vi "XYZ-IRC_Api.vi"(3 "精準度":dbl=30.0, 4 "ExitRange":dbl=0.08, 5 "加速度":dbl=800.0, 6 "目標電壓":dbl[](array[numeric])=[2.00487, 1.87997, 1.94422, 1.88569, 1.82844, 1.91098, 1.88335, 2.08625], 7 "最高速":dbl=1150.0, 8 "Error":errorcluster, 9 "副邊校正":T1(ring)=enum."無", 10 "主編校正":enum16{"前", "後", "オ", "右", "無"}(ring)=enum."無", 11 "X-Y-Z移動":dbl[](array[numeric])=[0.0, 0.0, 0.0]) -> (0 "Error Out":errorcluster)   [LabVIEW 2019]
uses:
  <vilib>/Platform/TimedLoop/XDataNode/timing_clust.ctl
  <vilib>/Platform/TimedLoop/XDataNode/nitl_modes.ctl
  <vilib>/Platform/TimedLoop/XDataNode/wakeup.ctl
  <vilib>/addons/control/pid/pid.llb/PID (DBL Array).vi
  <vilib>/platform/TimedLoop/XDataNode/XDataNode.xnode
  <vilib>/Platform/TimedLoop/XDataNode/XDNodeRunTimeDep.lvlib
  <vilib>/addons/control/pid/NI_PID_pid.lvlib
panel:
  in  "Stop":bool
  out "三角形?":bool
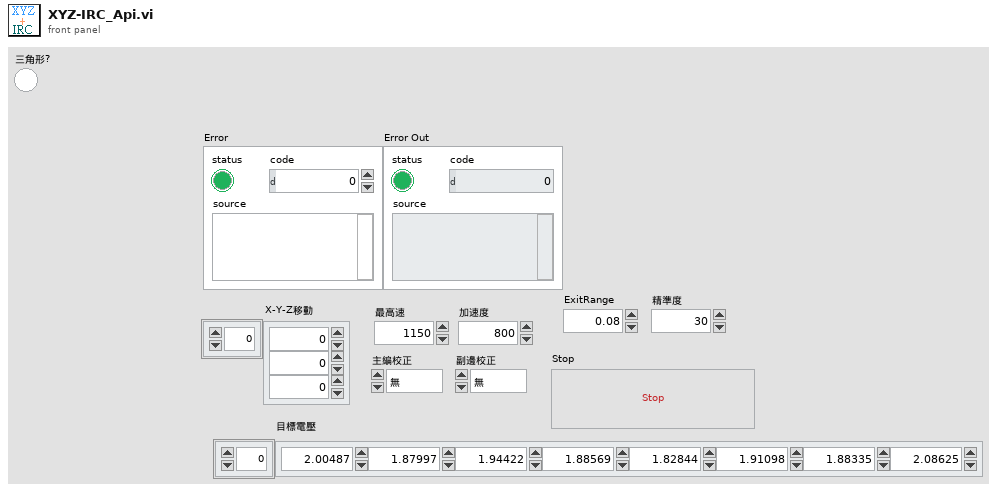
[diagram p1: front panel]
types:
  T1 = enum16{"前", "後", "オ", "右", "無", "0", "1", "2", "3", "4", "5", "6", "7"}
  T2 = cluster{"proportional gain (Kc)":dbl, "integral time (Ti, min)":dbl, "derivative time (Td, min)":dbl}[]
  T3 = typedef "XDNodeRunTimeDep.lvlib/timing_clust.ctl" = cluster{"Expected End [f-1]":u64, "Actual End [f-1]":u64, "Finished Late? [f-1]":bool, "Expected End [i-1]":u64, "Actual End [i-1]":u64, "Finished Late? [i-1]":bool, "Expected Start [i]":u64, "Actual Start [i]":u64, "Expected Start [f]":u64, "Actual Start [f]":u64, "Source Name":string, "Structure Name":string, "Period":i64, "Deadline":i64, "Offset":i64, "Start":i64, "Priority":i32, "Timeout":i32, "Mode":T4, "Wakeup Reason":T5, "Error":errorcluster, "Source Type":string, "Secondary Source Type":string, "Global End Time":u64, "Global Start Time":u64, "Frame Duration":u64, "Iteration Duration":u64, "Assigned CPU":i32, "I/O Scan Engine Mode":u32}
  T4 = typedef "XDNodeRunTimeDep.lvlib/nitl_modes.ctl" = enum32{"No Change", "Process missed periods, maintain original phase", "Discard missed periods, maintain original phase", "Process missed periods, ignore original phase", "Discard missed periods, ignore original phase"}
  T5 = typedef "XDNodeRunTimeDep.lvlib/wakeup.ctl" = enum32{"Normal", "Aborted", "Asynchronous wakeup", "Timing source error", "Timed loop error", "Timeout"}
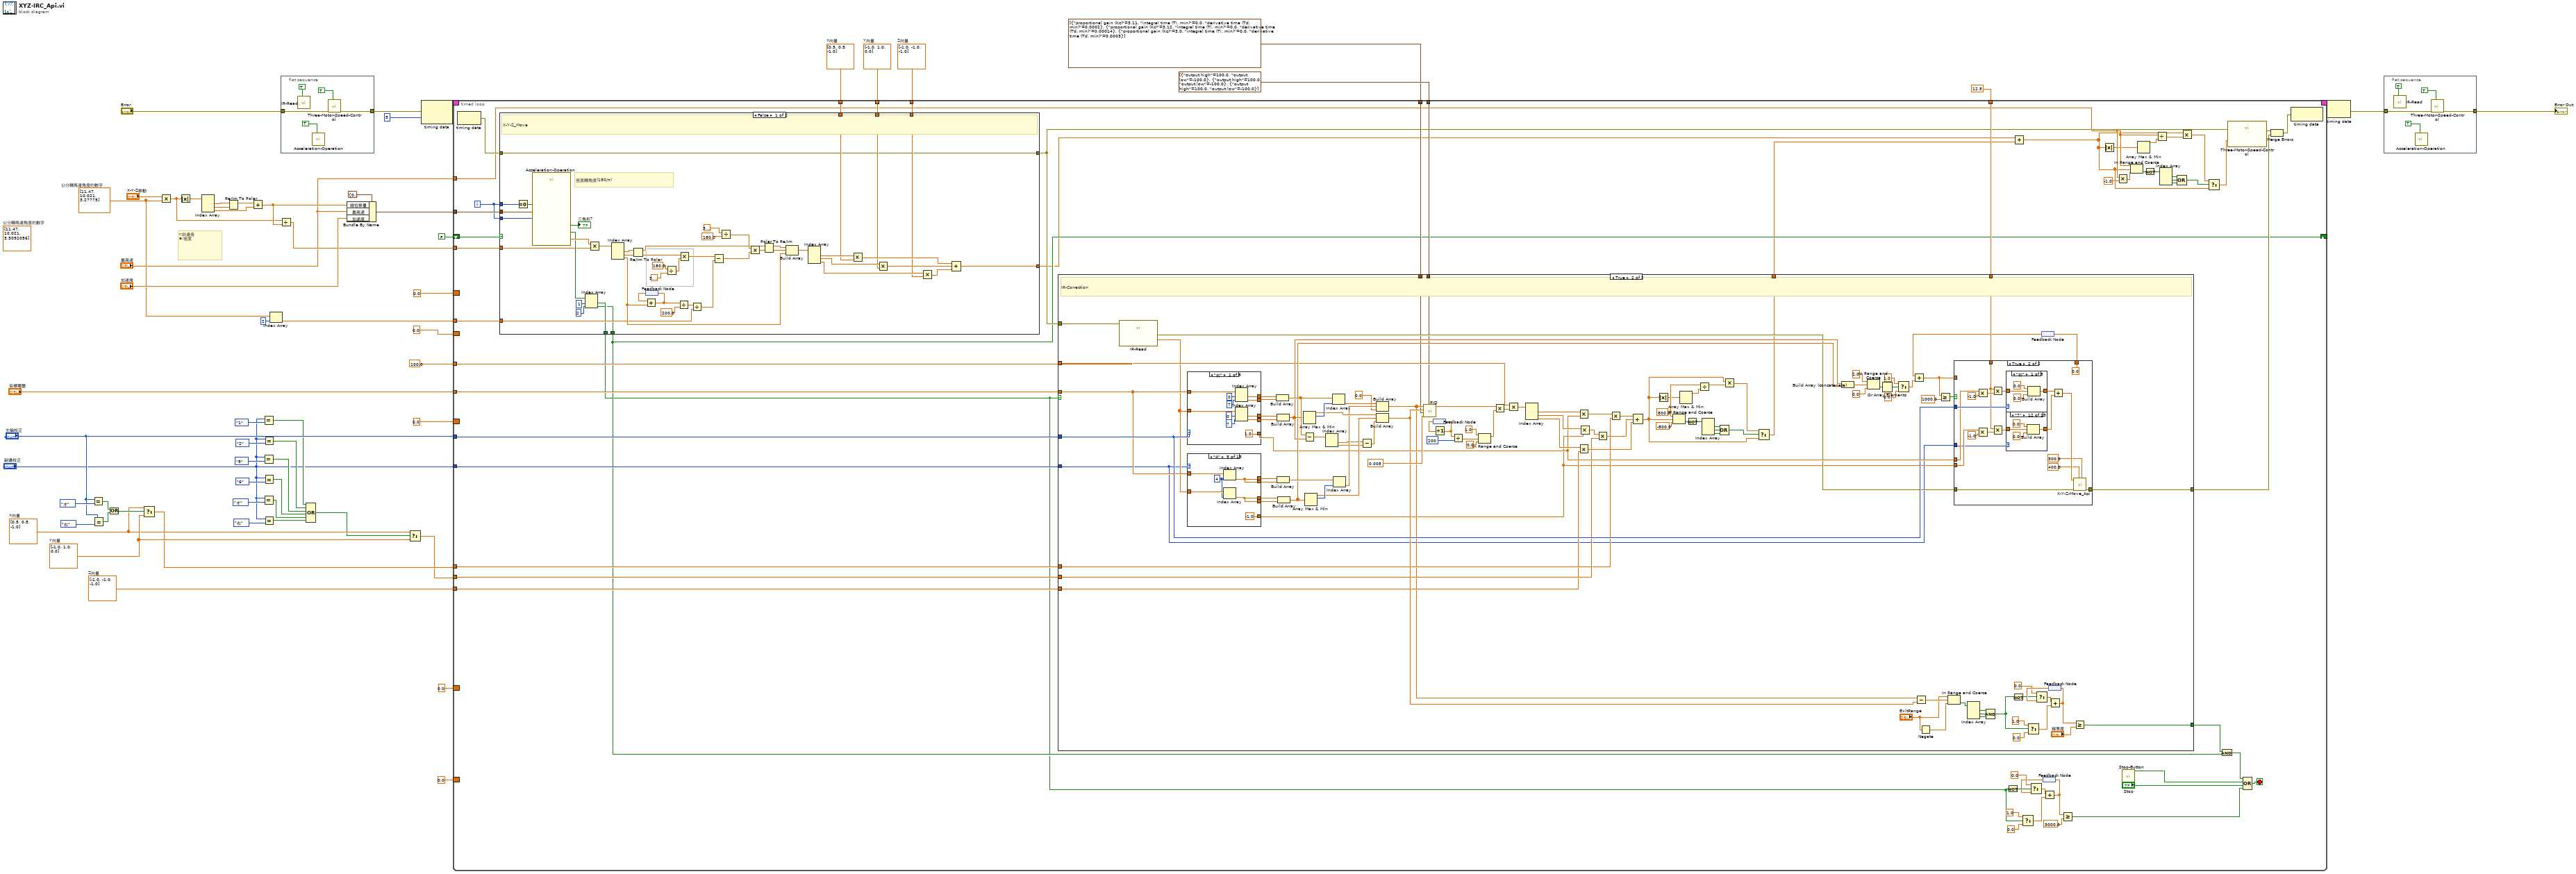
[diagram p0: block diagram]
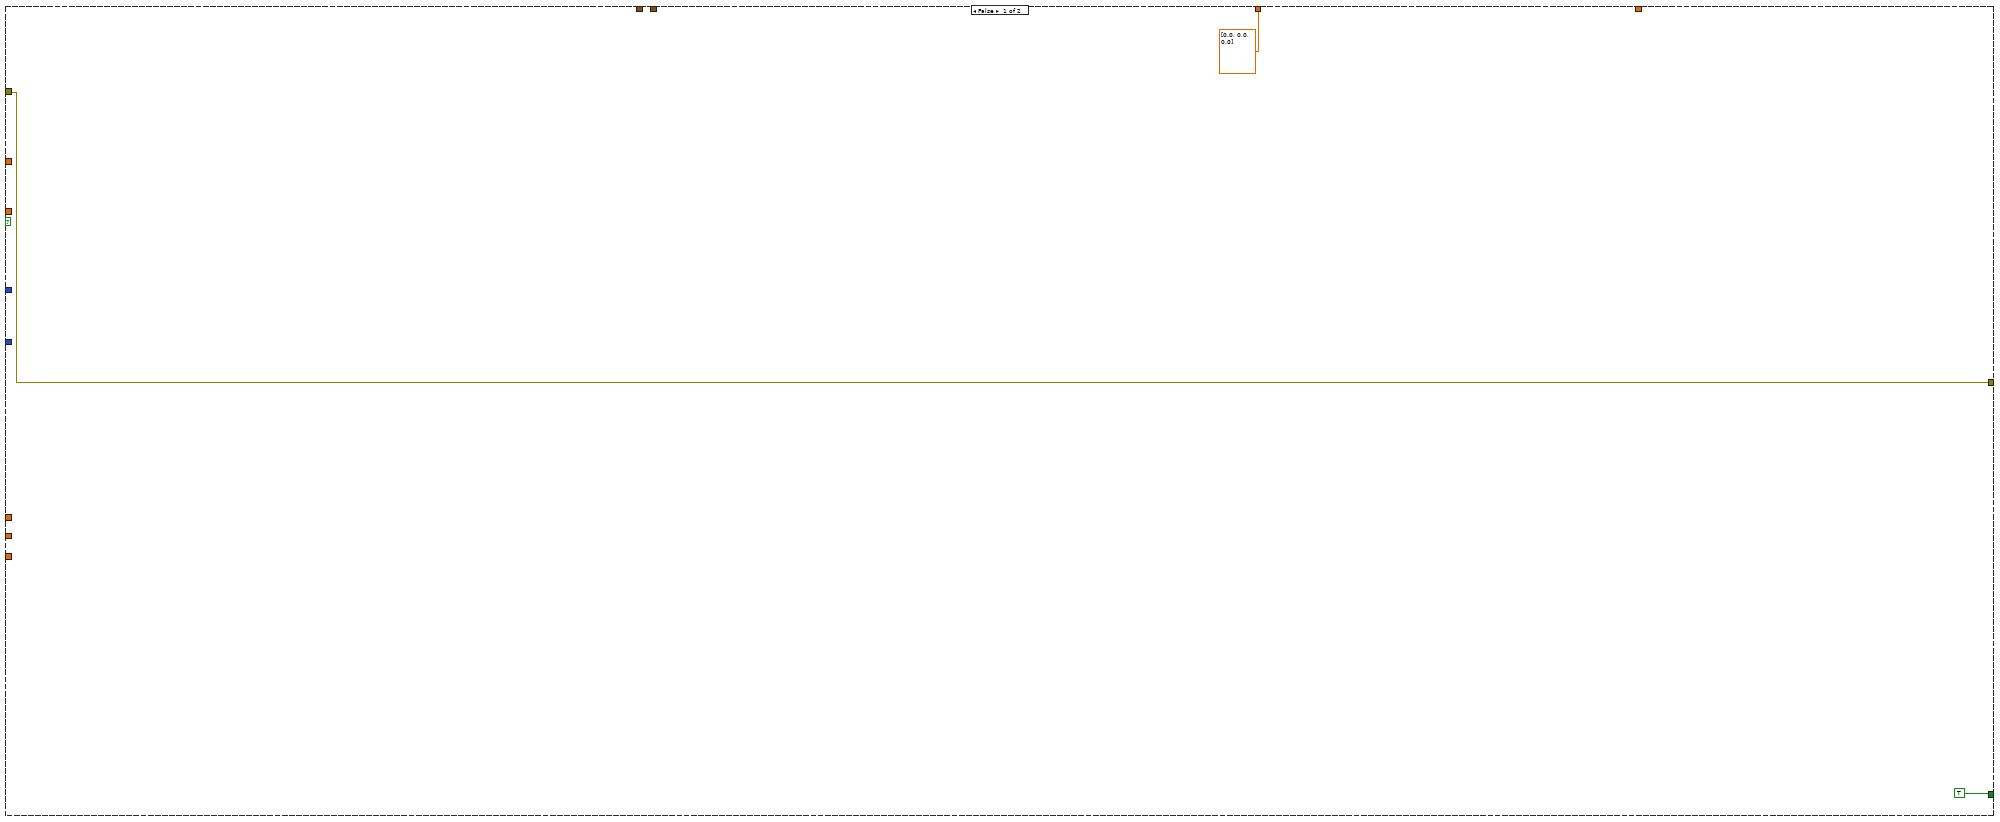
[diagram p2: hidden frame]
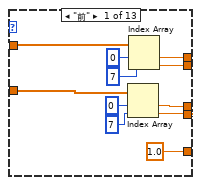
[diagram p3: hidden frame]
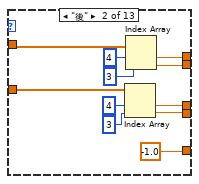
[diagram p4: hidden frame]
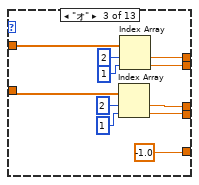
[diagram p5: hidden frame]
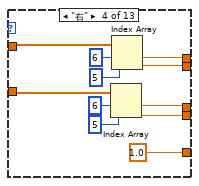
[diagram p6: hidden frame]
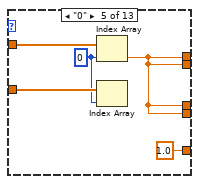
[diagram p7: hidden frame]
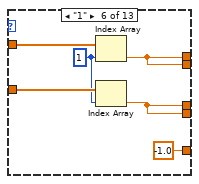
[diagram p8: hidden frame]
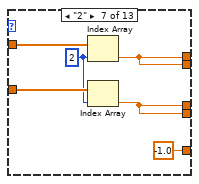
[diagram p9: hidden frame]
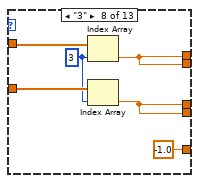
[diagram p10: hidden frame]
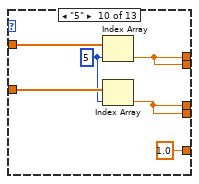
[diagram p11: hidden frame]
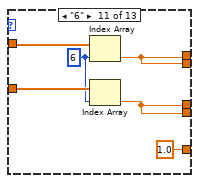
[diagram p12: hidden frame]
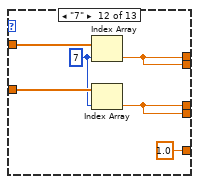
[diagram p13: hidden frame]
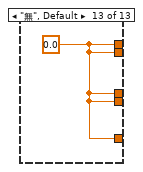
[diagram p14: hidden frame]
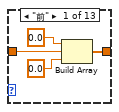
[diagram p16: hidden frame]
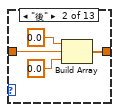
[diagram p17: hidden frame]
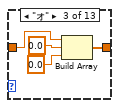
[diagram p18: hidden frame]
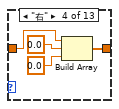
[diagram p19: hidden frame]
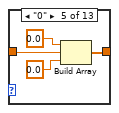
[diagram p20: hidden frame]
diagram:
  w25 = dbl[] [-1.0, -1.0, -1.0]  # Z向量
  w36 = dbl[] [-1.0, 1.0, 0.0]  # Y向量
  w35 = dbl[] [0.5, 0.5, -1.0]  # X向量
  w41 = dbl[] [-1.0, -1.0, -1.0]  # Z向量
  w42 = dbl[] [-1.0, 1.0, 0.0]  # Y向量
  w43 = dbl[] [0.5, 0.5, -1.0]  # X向量
  (unwired) dbl[] [11.47, 10.021, 3.3092056]  # 公分轉馬達角度的數字
  w49 = dbl[] [11.47, 10.021, 3.27775]  # 公分轉馬達角度的數字
  # "r:斜邊長\ne:徑度"
  n1 = Equal?(x="主編校正", y=enum16{"前", "後", "オ", "右", "無"}."オ") -> (x = y?=w38:bool)
  n2 = Equal?(x="主編校正", y=enum16{"前", "後", "オ", "右", "無"}."右") -> (x = y?=w39:bool)
  n3 = Or(x=w38, y=w39) -> (x .or. y?=w37:bool)
  n4 = Select(t=w35, s=w37, f=w36) -> (s? t:f=w27:dbl[])
  n5 = Multiply(x="X-Y-Z移動", y=w49) -> (x*y=w50:dbl[])
  n6 = Absolute Value(x=w50) -> (abs(x)=w58:dbl[])
  n7 = Index Array(array=w58) -> (element #1=w54:dbl, element #2=w59:dbl, element #3=w55:dbl)  [unwired: 3 in]
  n8 = Re/Im To Polar(2:w59, 3:w54) -> (1:w56:dbl)  [unwired: 1 out]
  n9 = Add(x=w56, y=w55) -> (x+y=w51:dbl)
  n10 = Equal?(x="副邊校正", y=T1."1") -> (x = y?=w5:bool)
  n11 = Equal?(x="副邊校正", y=T1."5") -> (x = y?=w4:bool)
  n12 = Equal?(x="副邊校正", y=T1."オ") -> (x = y?=w8:bool)
  n13 = Equal?(x="副邊校正", y=T1."2") -> (x = y?=w6:bool)
  n14 = Equal?(x="副邊校正", y=T1."6") -> (x = y?=w7:bool)
  n15 = Equal?(x="副邊校正", y=T1."右") -> (x = y?=w9:bool)
  n16 = Index Array(array=w49, index=2) -> (element=w45:dbl)
  n17 = Divide(x=w50, y=w51) -> (x/y=w46:dbl[])
  n18 = flat-sequence {
    tunnel: "Error" -> [w66]
    tunnel: [w65] -> w40
    frame #0 {
      n19 = call "IR-Read.vi"("Reset"=TRUE) -> ()  [unwired: 9 in, 2 out]
      n20 = call "Acceleration-Operation.vi"("Reset"=TRUE) -> ()  [unwired: 8 in, 3 out]
      n21 = call "Three-Motor-Speed-Control.vi"("Reset"=TRUE, "Error In"=w66) -> ("Error Out"=w65:errorcluster)  [unwired: 9 in]
    }
  }
  n22 = Compound Arithmetic op=OR(w5, w6, w4, w7, w8, w9) -> (w2:bool)
  n23 = Bundle By Name(cluster=cluster{"總位移量":dbl, "最高速":dbl, "加速度":dbl} {"總位移量"=0.0, "最高速"=0.0, "加速度"=0.0} ("計算設置"), "總位移量"=w51, "最高速"="最高速", "加速度"="加速度") -> (w47:cluster{"總位移量":dbl, "最高速":dbl, "加速度":dbl})
  n24 = Select(t=w35, s=w2, f=w36) -> (s? t:f=w26:dbl[])
  n25 = node-c288(w40, i64 5 ("Period")) -> (w62:T3)
  n26 = timed-loop {
    timing: w62 -> [_]
    timing-out: [_] -> w61
    tunnel: w47 -> [w123]
    tunnel: w46 -> [w122]
    tunnel: w45 -> [w121]
    border: 0.0 -> [_]
    tunnel: w43 -> [w120]
    tunnel: w42 -> [w119]
    tunnel: w41 -> [w118]
    tunnel: "目標電壓" -> [w112]
    tunnel: "主編校正" -> [w114]
    tunnel: "副邊校正" -> [w113]
    tunnel: 100.0 -> [w111]
    border: 0.0 -> [_]
    tunnel: 12.5 -> [w110]
    tunnel: w27 -> [w109]
    tunnel: w26 -> [w108]
    tunnel: w25 -> [w107]
    tunnel: cluster{"output high":dbl, "output low":dbl}[] [{"output high"=100.0, "output low"=-100.0}, {"output high"=100.0, "output low"=-100.0}, {"output high"=100.0, "output low"=-100.0}] ("output range") -> [w106]
    tunnel: T2 [{"proportional gain (Kc)"=3.11, "integral time (Ti, min)"=0.0, "derivative time (Td, min)"=0.0002}, {"proportional gain (Kc)"=3.12, "integral time (Ti, min)"=0.0, "derivative time (Td, min)"=0.00014}, {"proportional gain (Kc)"=3.0, "integral time (Ti, min)"=0.0, "derivative time (Td, min)"=0.0003}] ("PID gains") -> [w105]
    shift-right: [w98] -> _
    shift-left: FALSE -> [w97]
    border: 0.0 -> [_]
    tunnel: "最高速" -> [w82]
    border: 0.0 -> [_]
    border: 0.0 -> [_]
    i -> [w103]
    stop <- w115 stop-if-true
    n27 = node-c288() -> (w124:errorcluster)  [unwired: 1 in]
    n28 = case shown="False" w97 {
      tunnel: w124 -> [w466 w509]
      tunnel: w103 -> [w474 _]
      tunnel: w123 -> [w473 _]
      tunnel: w122 -> [w472 _]
      tunnel: w121 -> [w471 _]
      tunnel: w120 -> [w470 _]
      tunnel: w119 -> [w469 _]
      tunnel: w118 -> [w468 _]
      tunnel: [w467 dbl[] [0.0, 0.0, 0.0]] -> w96
      tunnel: [w466 w509] -> w99
      tunnel: [w463 w508] -> w69
      tunnel: w103 -> [w465 _]
      tunnel: [w461 w508] -> w98
      frame False {
        # "徑度轉角度(180/π)"
        # "X-Y-Z_Move"
        n29 = Equal To 0?(x=w474) -> (x = 0?=w506:bool)
        n30 = call "Acceleration-Operation.vi"("Reset"=w506, "迴圈( I )"=w465, "計算設置"=w473) -> ("完成?"=w504:bool[], "速度"=w507:dbl, "三角形?"=→"三角形?":bool)  [unwired: 6 in]
        n31 = Index Array(array=w504, index #1=1 ("index"), index #2=2 ("index")) -> (element #1=w463:bool, element #2=w461:bool)
        n32 = Multiply(x=w507, y=w472) -> (x*y=w503:dbl[])
        n33 = Index Array(array=w503) -> (element #1=w502:dbl, element #2=w501:dbl, element #3=w484:dbl)  [unwired: 3 in]
        n34 = Re/Im To Polar(2:w501, 3:w502) -> (0:w500:dbl, 1:w487:dbl)
        n35 = feedback #1() -> (w496:dbl)
        n36 = Add(x=w496, y=w484) -> (x+y=w495:dbl)
        n37 = feedback-in #1(w495) -> ()
        n38 = Divide(x=180.0, y=3.141592653589793) -> (x/y=w497:dbl)
        n39 = Divide(x=w495, y=200.0) -> (x/y=w476:dbl)
        n40 = Multiply(x=w500, y=w497) -> (x*y=w493:dbl)
        n41 = Divide(x=w476, y=w471) -> (x/y=w475:dbl)
        n42 = Subtract(x=w493, y=w475) -> (x-y=w489:dbl)
        n43 = Divide(x=3.141592653589793, y=180.0 ("x")) -> (x/y=w490:dbl)
        n44 = Multiply(x=w490, y=w489) -> (x*y=w488:dbl)
        n45 = Polar To Re/Im(2:w488, 3:w487) -> (0:w485:dbl, 1:w486:dbl)
        n46 = Build Array(w486, w485, w484) -> (w483:dbl[])
        n47 = Index Array(array=w483) -> (element #1=w482:dbl, element #2=w481:dbl, element #3=w480:dbl)  [unwired: 3 in]
        n48 = Multiply(x=w482, y=w470) -> (x*y=w479:dbl[])
        n49 = Multiply(x=w481, y=w469) -> (x*y=w478:dbl[])
        n50 = Multiply(x=w480, y=w468) -> (x*y=w477:dbl[])
        n51 = Compound Arithmetic op=ADD(w479, w478, w477) -> (w467:dbl[])
      }
      frame True {
        w508 = TRUE
      }
    }
    n52 = case shown="True" w69 {
      tunnel: w99 -> [w127 w186]
      tunnel: w111 -> [_ w185]
      tunnel: w114 -> [_ w184]
      tunnel: w113 -> [_ w133]
      tunnel: w112 -> [_ w135]
      tunnel: w110 -> [_ w175]
      tunnel: [dbl[] [0.0, 0.0, 0.0] w173] -> w95
      tunnel: [w127 w172] -> w100
      tunnel: w109 -> [_ w170]
      tunnel: w108 -> [_ w171]
      tunnel: w107 -> [_ w169]
      tunnel: w106 -> [_ w167]
      tunnel: w105 -> [_ w166]
      tunnel: [TRUE w140] -> w83
      frame False {
      }
      frame True {
        w131 = 800.0
        # "IR-Correction"
        n53 = call "IR-Read.vi"("Error In"=w186) -> ("Error Out"=w174:errorcluster, "輸出紅外線值"=w134:dbl[])  [unwired: 9 in]
        n54 = case shown="\"前\"" w184 {
          tunnel: w135 -> [w422 w428 w439 w455 _]
          tunnel: w134 -> [w421 w427 w438 w451 _]
          tunnel: [w420 w429 w444 w449 w460] -> w232
          tunnel: [w419 w430 w443 w450 w460] -> w231
          tunnel: [w418 w431 w442 w452 w460] -> w230
          tunnel: [w417 w432 w441 w453 w460] -> w229
          tunnel: [1.0 ("y") -1.0 ("y") -1.0 ("y") 1.0 ("y") w460] -> w187
          frame "前" {
            n55 = Index Array(array=w421, index #1=0 ("index"), index #2=7 ("index")) -> (element #1=w418:dbl, element #2=w417:dbl)
            n56 = Index Array(array=w422, index #1=0 ("index"), index #2=7 ("index")) -> (element #1=w420:dbl, element #2=w419:dbl)
          }
          frame "後" {
            n57 = Index Array(array=w427, index #1=4 ("index"), index #2=3 ("index")) -> (element #1=w431:dbl, element #2=w432:dbl)
            n58 = Index Array(array=w428, index #1=4 ("index"), index #2=3 ("index")) -> (element #1=w429:dbl, element #2=w430:dbl)
          }
          frame "オ" {
            n59 = Index Array(array=w438, index #1=2 ("index"), index #2=1 ("index")) -> (element #1=w442:dbl, element #2=w441:dbl)
            n60 = Index Array(array=w439, index #1=2 ("index"), index #2=1 ("index")) -> (element #1=w444:dbl, element #2=w443:dbl)
          }
          frame "右" {
            n61 = Index Array(array=w451, index #1=6 ("index"), index #2=5 ("index")) -> (element #1=w452:dbl, element #2=w453:dbl)
            n62 = Index Array(array=w455, index #1=6 ("index"), index #2=5 ("index")) -> (element #1=w449:dbl, element #2=w450:dbl)
          }
          frame "無", Default {
            w460 = 0.0 ("Numeric")
          }
        }
        n63 = case shown="\"4\"" w133 {
          tunnel: w135 -> [w239 w245 w259 w272 w281 w287 w293 w299 w305 w311 w317 w323 _]
          tunnel: w134 -> [w238 w244 w260 w271 w278 w284 w291 w297 w303 w308 w314 w321 _]
          tunnel: [w237 w246 w262 w270 w280 w286 w290 w295 w301 w310 w316 w319 w324] -> w139
          tunnel: [w236 w247 w256 w269 w280 w286 w290 w295 w301 w310 w316 w319 w324] -> w138
          tunnel: [w235 w248 w261 w268 w280 w282 w289 w294 w300 w306 w312 w318 w324] -> w137
          tunnel: [w234 w249 w255 w267 w280 w282 w289 w294 w300 w306 w312 w318 w324] -> w136
          tunnel: [1.0 ("y") -1.0 ("y") -1.0 ("y") 1.0 ("y") 1.0 ("Numeric") -1.0 ("Numeric") -1.0 ("Numeric") -1.0 ("Numeric") -1.0 ("Numeric") 1.0 ("Numeric") 1.0 ("Numeric") 1.0 ("Numeric") w324] -> w132
          frame "前" {
            n64 = Index Array(array=w238, index #1=0 ("index"), index #2=7 ("index")) -> (element #1=w235:dbl, element #2=w234:dbl)
            n65 = Index Array(array=w239, index #1=0 ("index"), index #2=7 ("index")) -> (element #1=w237:dbl, element #2=w236:dbl)
          }
          frame "後" {
            n66 = Index Array(array=w244, index #1=4 ("index"), index #2=3 ("index")) -> (element #1=w248:dbl, element #2=w249:dbl)
            n67 = Index Array(array=w245, index #1=4 ("index"), index #2=3 ("index")) -> (element #1=w246:dbl, element #2=w247:dbl)
          }
          frame "オ" {
            n68 = Index Array(array=w260, index #1=2 ("index"), index #2=1 ("index")) -> (element #1=w261:dbl, element #2=w255:dbl)
            n69 = Index Array(array=w259, index #1=2 ("index"), index #2=1 ("index")) -> (element #1=w262:dbl, element #2=w256:dbl)
          }
          frame "右" {
            n70 = Index Array(array=w271, index #1=6 ("index"), index #2=5 ("index")) -> (element #1=w268:dbl, element #2=w267:dbl)
            n71 = Index Array(array=w272, index #1=6 ("index"), index #2=5 ("index")) -> (element #1=w270:dbl, element #2=w269:dbl)
          }
          frame "0" {
            w277 = 0 ("index")
            n72 = Index Array(array=w281, index=w277) -> (element=w280:dbl)
            n73 = Index Array(array=w278, index=w277) -> ()  [unwired: 1 out]
          }
          frame "1" {
            w283 = 1 ("index")
            n74 = Index Array(array=w287, index=w283) -> (element=w286:dbl)
            n75 = Index Array(array=w284, index=w283) -> (element=w282:dbl)
          }
          frame "2" {
            w288 = 2 ("index")
            n76 = Index Array(array=w293, index=w288) -> (element=w290:dbl)
            n77 = Index Array(array=w291, index=w288) -> (element=w289:dbl)
          }
          frame "3" {
            w296 = 3 ("index")
            n78 = Index Array(array=w299, index=w296) -> (element=w295:dbl)
            n79 = Index Array(array=w297, index=w296) -> (element=w294:dbl)
          }
          frame "4" {
            w302 = 4 ("index")
            n80 = Index Array(array=w305, index=w302) -> (element=w301:dbl)
            n81 = Index Array(array=w303, index=w302) -> (element=w300:dbl)
          }
          frame "5" {
            w307 = 5 ("index")
            n82 = Index Array(array=w311, index=w307) -> (element=w310:dbl)
            n83 = Index Array(array=w308, index=w307) -> (element=w306:dbl)
          }
          frame "6" {
            w313 = 6 ("index")
            n84 = Index Array(array=w317, index=w313) -> (element=w316:dbl)
            n85 = Index Array(array=w314, index=w313) -> (element=w312:dbl)
          }
          frame "7" {
            w320 = 7 ("index")
            n86 = Index Array(array=w323, index=w320) -> (element=w319:dbl)
            n87 = Index Array(array=w321, index=w320) -> (element=w318:dbl)
          }
          frame "無", Default {
            w324 = 0.0 ("Numeric")
          }
        }
        n88 = Build Array(w232, w231) -> (w220:dbl[])
        n89 = Build Array(w230, w229) -> (w189:dbl[])
        n90 = Build Array(w139, w138) -> (w224:dbl[])
        n91 = Build Array(w137, w136) -> (w188:dbl[])
        n92 = Array Max & Min(array=w189) -> (max value=w226:dbl, max index (indices)=w228:i32)  [unwired: 2 out]
        n93 = Subtract(x=w220, y=w189) -> (x-y=w219:dbl[])
        n94 = Array Max & Min(array=w188) -> (max value=w222:dbl, max index (indices)=w225:i32)  [unwired: 2 out]
        n95 = Index Array(array=w219) -> (element #1=w218:dbl, element #2=w217:dbl)  [unwired: 2 in]
        n96 = Index Array(array=w220, index=w228) -> (element=w227:dbl)
        n97 = Index Array(array=w224, index=w225) -> (element=w223:dbl)
        n98 = Subtract(x=w218, y=w217) -> (x-y=w216:dbl)
        n99 = Build Array(w227, w223, 0.0 ("element")) -> (w168:dbl[])
        n100 = Build Array(w226, w222, w216) -> (w176:dbl[])
        n101 = call-poly <vilib>:"PID.vi"("output range"=w167, "dt (s)"=0.005, "PID gains"=w166, "process variable"=w176, "setpoint"=w168) -> ("output"=w193:dbl[])  [unwired: 5 in, 1 out]
        n102 = feedback #2() -> (w165:dbl)
        n103 = Increment(x=w165) -> (x+1=w164:dbl)
        n104 = feedback-in #2(w164) -> ()
        n105 = Divide(x=w164, y=200) -> (x/y=w197:dbl)
        n106 = In Range and Coerce(upper limit=1.0, x=w197, lower limit=0.0) -> (coerced(x)=w194:dbl)  [unwired: 1 out]
        n107 = Multiply(x=w193, y=w194) -> (x*y=w191:dbl[])
        n108 = Multiply(x=w185, y=w191) -> (x*y=w192:dbl[])
        n109 = Index Array(array=w192) -> (element #1=w214:dbl, element #2=w213:dbl, element #3=w210:dbl)  [unwired: 3 in]
        n110 = Multiply(x=w214, y=w187) -> (x*y=w212:dbl)
        n111 = Multiply(x=w210, y=w169) -> (x*y=w207:dbl[])
        n112 = Multiply(x=w213, y=w132) -> (x*y=w211:dbl)
        n113 = Multiply(x=w211, y=w171) -> (x*y=w208:dbl[])
        n114 = Multiply(x=w212, y=w170) -> (x*y=w209:dbl[])
        n115 = Compound Arithmetic op=ADD(w209, w208, w207) -> (w129:dbl[])
        n116 = Absolute Value(x=w129) -> (abs(x)=w130:dbl[])
        n117 = In Range and Coerce(upper limit=w131, x=w129, lower limit=-800.0) -> (In Range?=w205:bool[])  [unwired: 1 out]
        n118 = Array Max & Min(array=w130) -> (max value=w190:dbl)  [unwired: 3 out]
        n119 = Not(x=w205) -> (.not. x?=w204:bool[])
        n120 = Divide(x=w131, y=w190) -> (x/y=w200:dbl)
        n121 = Index Array(array=w204) -> (element #1=w203:bool, element #2=w128:bool, element #3=w202:bool)  [unwired: 3 in]
        n122 = Compound Arithmetic op=OR(w203, w128, w202) -> (w201:bool)
        n123 = Multiply(x=w129, y=w200) -> (x*y=w199:dbl[])
        n124 = Select(t=w199, s=w201, f=w129) -> (s? t:f=w173:dbl[])
        n125 = Build Array (concatenate)(w189, w188) -> (w163:dbl[])
        n126 = In Range and Coerce(upper limit=2.0 ("dt (s)"), x=w163, lower limit=0.0 ("dt (s)")) -> (In Range?=w160:bool[])  [unwired: 1 out]
        n127 = Or Array Elements(Boolean array=w160) -> (logical OR=w159:bool)
        n128 = Select(t=1.0, s=w159, f=0.0 ("t")) -> (s? t:f=w156:dbl)
        n129 = Subtract(x=w168, y=w176) -> (x-y=w183:dbl[])
        n130 = Negate(x="ExitRange") -> (-x=w178:dbl)
        n131 = In Range and Coerce(upper limit="ExitRange", x=w183, lower limit=w178) -> (In Range?=w182:bool[])  [unwired: 1 out]
        n132 = Index Array(array=w182) -> (element #1=w181:bool, element #2=w180:bool, element #3=w179:bool)  [unwired: 3 in]
        n133 = Compound Arithmetic op=AND(w181, w180, w179) -> (w141:bool)
        n134 = Not(x=w141) -> (.not. x?=w146:bool)
        n135 = Select(t=1.0, s=w141, f=0.0) -> (s? t:f=w148:dbl)
        n136 = feedback #3() -> (w154:dbl)
        n137 = Add(x=w154, y=w156) -> (x+y=w153:dbl)
        n138 = Greater Or Equal?(x=w153, y=1000.0) -> (x >= y?=w151:bool)
        n139 = case shown="True" w151 {
          tunnel: [w326 0.0] -> w155
          tunnel: w153 -> [w326 _]
          tunnel: w174 -> [w325 w344]
          tunnel: [w325 w343] -> w172
          tunnel: w184 -> [_ w342]
          tunnel: w133 -> [_ w328]
          tunnel: w175 -> [_ w334]
          tunnel: w187 -> [_ w340]
          tunnel: w132 -> [_ w335]
          frame False {
          }
          frame True {
            n140 = Multiply(x=w340, y=-1.0) -> (x*y=w341:dbl)
            n141 = Multiply(x=w335, y=-1.0) -> (x*y=w336:dbl)
            n142 = Multiply(x=w334, y=w341) -> (x*y=w338:dbl)
            n143 = Multiply(x=w334, y=w336) -> (x*y=w329:dbl)
            n144 = case shown="\"前\"" w342 {
              tunnel: w338 -> [w400 w404 w406 w410 _]
              tunnel: [w397 w401 w405 w409 w413] -> w333
              frame "前" {
                n145 = Build Array(0.0 ("element"), w400, 0.0 ("element")) -> (w397:dbl[])
              }
              frame "後" {
                n146 = Build Array(0.0 ("element"), w404, 0.0 ("element")) -> (w401:dbl[])
              }
              frame "オ" {
                n147 = Build Array(w406, 0.0 ("element"), 0.0 ("element")) -> (w405:dbl[])
              }
              frame "右" {
                n148 = Build Array(w410, 0.0 ("element"), 0.0 ("element")) -> (w409:dbl[])
              }
              frame "無", Default {
                w414 = 0.0 ("element")
                n149 = Build Array(w414, w414, 0.0 ("element")) -> (w413:dbl[])
              }
            }
            n150 = case shown="\"7\"" w328 {
              tunnel: w329 -> [w349 w353 w354 w358 w363 w367 w370 w375 w379 w382 w386 w390 _]
              tunnel: [w346 w350 w355 w359 w362 w366 w371 w374 w378 w383 w387 w391 w394] -> w327
              frame "前" {
                n151 = Build Array(0.0 ("element"), w349, 0.0 ("element")) -> (w346:dbl[])
              }
              frame "後" {
                n152 = Build Array(0.0 ("element"), w353, 0.0 ("element")) -> (w350:dbl[])
              }
              frame "オ" {
                n153 = Build Array(w354, 0.0 ("element"), 0.0 ("element")) -> (w355:dbl[])
              }
              frame "右" {
                n154 = Build Array(w358, 0.0 ("element"), 0.0 ("element")) -> (w359:dbl[])
              }
              frame "0" {
                n155 = Build Array(0.0 ("element"), w363, 0.0 ("element")) -> (w362:dbl[])
              }
              frame "1" {
                n156 = Build Array(w367, 0.0 ("element"), 0.0 ("element")) -> (w366:dbl[])
              }
              frame "2" {
                n157 = Build Array(w370, 0.0 ("element"), 0.0 ("element")) -> (w371:dbl[])
              }
              frame "3" {
                n158 = Build Array(0.0 ("element"), w375, 0.0 ("element")) -> (w374:dbl[])
              }
              frame "4" {
                n159 = Build Array(0.0 ("element"), w379, 0.0 ("element")) -> (w378:dbl[])
              }
              frame "5" {
                n160 = Build Array(w382, 0.0 ("element"), 0.0 ("element")) -> (w383:dbl[])
              }
              frame "6" {
                n161 = Build Array(w386, 0.0 ("element"), 0.0 ("element")) -> (w387:dbl[])
              }
              frame "7" {
                n162 = Build Array(0.0 ("element"), w390, 0.0 ("element")) -> (w391:dbl[])
              }
              frame "無", Default {
                w395 = 0.0 ("element")
                n163 = Build Array(w395, w395, 0.0 ("element")) -> (w394:dbl[])
              }
            }
            n164 = Add(x=w333, y=w327) -> (x+y=w332:dbl[])
            n165 = call "X-Y-Z-Move_Api.vi"("加速度"=300.0, "最高速"=400.0, "Error In"=w344, "X-Y-Z移動"=w332) -> ("Error Out"=w343:errorcluster)  [unwired: 6 in, 1 out]
          }
        }
        n166 = feedback-in #3(w155) -> ()
        n167 = feedback #4() -> (w147:dbl)
        n168 = Select(t=0.0, s=w146, f=w147) -> (s? t:f=w144:dbl)
        n169 = Add(x=w144, y=w148) -> (x+y=w143:dbl)
        n170 = feedback-in #4(w143) -> ()
        n171 = Greater Or Equal?(x=w143, y="精準度") -> (x >= y?=w140:bool)
      }
    }
    n172 = Not(x=w69) -> (.not. x?=w74:bool)
    n173 = Add(x=w96, y=w95) -> (x+y=w79:dbl[])
    n174 = Select(t=1.0, s=w69, f=0.0) -> (s? t:f=w72:dbl)
    n175 = feedback #5() -> (w73:dbl)
    n176 = Select(t=0.0, s=w74, f=w73) -> (s? t:f=w76:dbl)
    n177 = Add(x=w76, y=w72) -> (x+y=w77:dbl)
    n178 = feedback-in #5(w77) -> ()
    n179 = Greater Or Equal?(x=w77, y=3000.0) -> (x >= y?=w68:bool)
    n180 = Absolute Value(x=w79) -> (abs(x)=w80:dbl[])
    n181 = Multiply(x=w82, y=-1.0) -> (x*y=w85:dbl)
    n182 = call "Stop-Button.vi"() -> ("顯示按下?"=w117:bool)  [unwired: 10 in, 1 out]
    n183 = In Range and Coerce(upper limit=w82, x=w79, lower limit=w85) -> (In Range?=w94:bool[])  [unwired: 1 out]
    n184 = Array Max & Min(array=w80) -> (max value=w86:dbl)  [unwired: 3 out]
    n185 = Not(x=w94) -> (.not. x?=w93:bool[])
    n186 = Divide(x=w82, y=w86) -> (x/y=w88:dbl)
    n187 = Index Array(array=w93) -> (element #1=w92:bool, element #2=w91:bool, element #3=w90:bool)  [unwired: 3 in]
    n188 = Compound Arithmetic op=OR(w92, w91, w90) -> (w89:bool)
    n189 = Multiply(x=w79, y=w88) -> (x*y=w87:dbl[])
    n190 = Select(t=w87, s=w89, f=w79) -> (s? t:f=w81:dbl[])
    n191 = And(x=w83, y=w98) -> (x .and. y?=w104:bool)
    n192 = call "Three-Motor-Speed-Control.vi"("Error In"=w99, "速度(秒/度)"=w81) -> ("Error Out"=w102:errorcluster)  [unwired: 9 in]
    n193 = Compound Arithmetic op=OR(w104, w117, "Stop", w68) -> (w115:bool)
    n194 = Merge Errors(w102, w100) -> (w101:errorcluster)
    n195 = node-c288(w101) -> ()  [unwired: 1 out]
  }
  n196 = node-c288(w61) -> (w22:errorcluster)
  n197 = flat-sequence {
    tunnel: w22 -> [w519]
    tunnel: [w518] -> w18
    frame #0 {
      n198 = call "IR-Read.vi"("Reset"=TRUE) -> ()  [unwired: 9 in, 2 out]
      n199 = call "Acceleration-Operation.vi"("Reset"=TRUE) -> ()  [unwired: 8 in, 3 out]
      n200 = call "Three-Motor-Speed-Control.vi"("Reset"=TRUE, "Error In"=w519) -> ("Error Out"=w518:errorcluster)  [unwired: 9 in]
    }
  }
  "Error Out" <- w18
